vi "decimal_to_bits_att.vi"(2 "attenuation decimal":u8=15, 3 "error in":errorcluster) -> (0 "attenuation binary":string, 1 "error out":errorcluster)   [LabVIEW 2021]
panel:
  out "Byte Binary Rep.":string
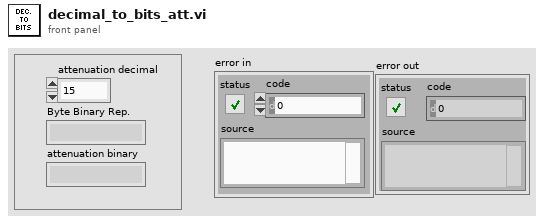
[diagram p1: front panel]
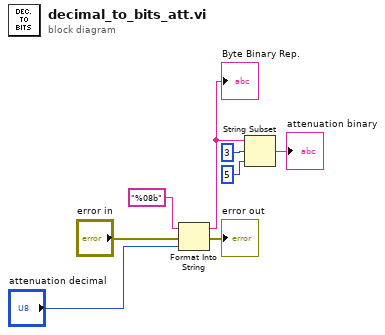
[diagram p0: block diagram]
diagram:
  n1 = Format Into String(format string="%08b", error in="error in", "attenuation decimal") -> (resulting string=w3:string, error out=→"error out":errorcluster)  [unwired: 1 in]
  "Byte Binary Rep." <- w3
  n2 = String Subset(string=w3, offset (0)=3, length (rest)=5 ("length (rest)")) -> (substring=→"attenuation binary":string)
